vi "Create PyObject.vi"(8 "error in (no error)":errorcluster, 9 "Methods":T1[](array[typedef]), 10 "PyObject Name":string, 11 "Node in":refnum<class "PyObject.lvclass">) -> (0 "error out":errorcluster, 3 "Node out":refnum<class "PyObject.lvclass">)   [LabVIEW 2015, in "JKI_Python_Bridge_for_LV.lvlib" / "PyObject.lvclass"]
uses:
  PyObject.lvclass
  TypeDefs/PyObject Method.ctl
  TypeDefs/Private Data.ctl
  Server/Type Definitions/Python Method Call - Event Registration.ctl
  Call/Call.lvclass
  Server/Type Definitions/Public Events - Cluster.ctl
  PyObject.lvclass/PyObject.ctl
  Server/Server.lvclass
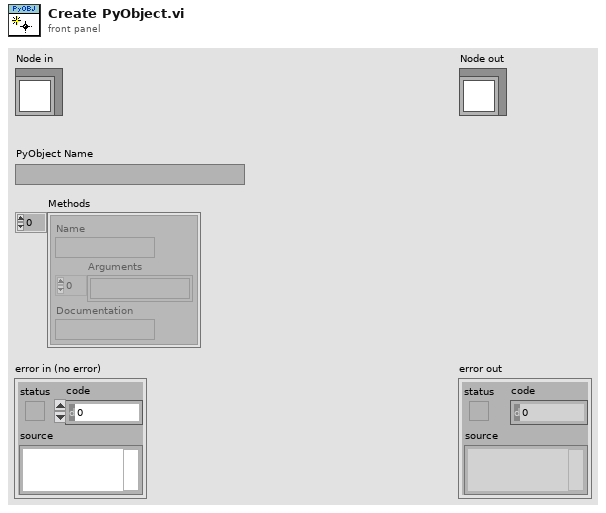
[diagram p1: front panel]
types:
  T1 = typedef "JKI_Python_Bridge_for_LV.lvlib/PyObject.lvclass/PyObject Method.ctl" = cluster{"Name":string, "Arguments":string[], "Documentation":string}
  T2 = typedef "JKI_Python_Bridge_for_LV.lvlib/PyObject.lvclass/Private Data.ctl" = cluster{"Call Registration":T3, "Functions":T1[], "Object Name":string}
  T3 = typedef "JKI_Python_Bridge_for_LV.lvlib/Server.lvclass/Python Method Call - Event Registration.ctl" = refnum<event-registration>
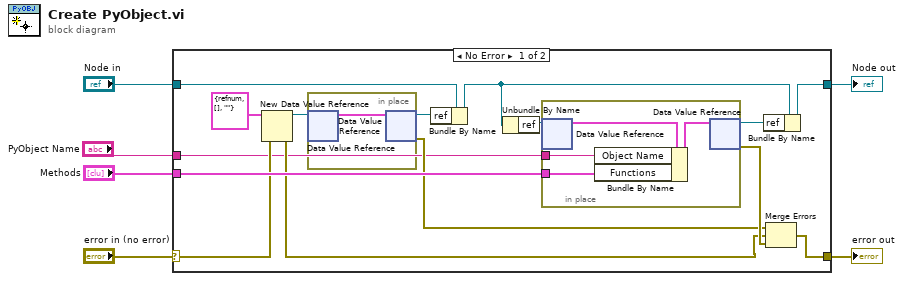
[diagram p0: block diagram]
diagram:
  n1 = case shown="No Error" "error in (no error)" {
    selector: "error in (no error)" -> [w15 w27]
    tunnel: [w8 w27] -> w5
    tunnel: [w20 w28] -> w3
    tunnel: "Node in" -> [w14 w28]
    tunnel: "Methods" -> [w18 _]
    tunnel: "PyObject Name" -> [w7 _]
    frame No Error {
      n2 = New Data Value Reference(data value=T2 {"Call Registration"=refnum, "Functions"=[], "Object Name"=""} ("Private Data"), error in=w15) -> (data value reference=w17:refnum<data-value>, error out=w9:errorcluster)
      n3 = in-place {
        n4 = in-place-dvr #1(w17) -> (w22:T2)  [unwired: 1 out]
        n5 = in-place-dvr #1(w22) -> (w12:refnum<data-value>, w10:errorcluster)
      }
      n6 = Bundle By Name(cluster=w14, "ref"=w12) -> (w13:refnum<class "PyObject.lvclass">)
      n7 = Unbundle By Name(w13) -> ("ref"=w21:refnum<data-value>)
      n8 = in-place {
        in-place-border: w18 -> [w24]
        in-place-border: w7 -> [w23]
        n9 = in-place-dvr #2(w21) -> (w26:T2)  [unwired: 1 out]
        n10 = Bundle By Name(cluster=w26, "Object Name"=w23, "Functions"=w24) -> (w25:T2)
        n11 = in-place-dvr #2(w25) -> (w19:refnum<data-value>, w11:errorcluster)
      }
      n12 = Bundle By Name(cluster=w13, "ref"=w19) -> (w20:refnum<class "PyObject.lvclass">)
      n13 = Merge Errors(w10, w9, w11) -> (w8:errorcluster)
    }
    frame Error {
    }
  }
  "error out" <- w5
  "Node out" <- w3
